vi "Read series.vi"(8 "error in (no error)":errorcluster, 11 "InovanceModbusTcp in":refnum<class "DeltaTcp.lvclass">) -> (0 "error out":errorcluster, 2 "series":i32(ring)=2 items=["DVP", "AS"], 3 "InovanceModbusTcp out":refnum<class "DeltaTcp.lvclass">)   [LabVIEW 2020, in "HslCommunication.lvlib" / "DeltaTcp.lvclass"]
uses:
  DeltaTcp.lvclass
  DeltaTcp.lvclass/DeltaTcp.ctl
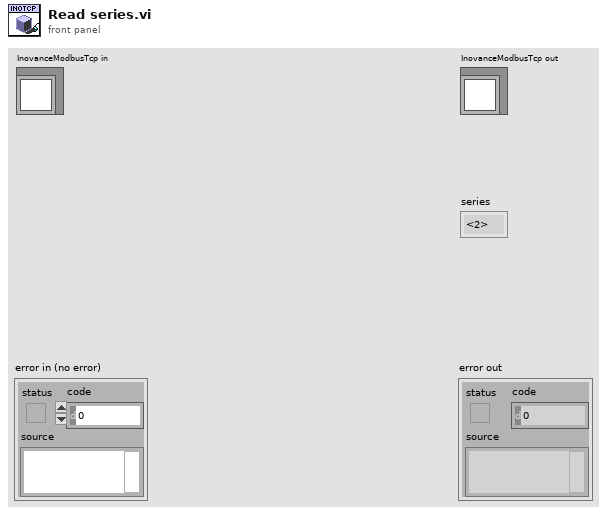
[diagram p1: front panel]
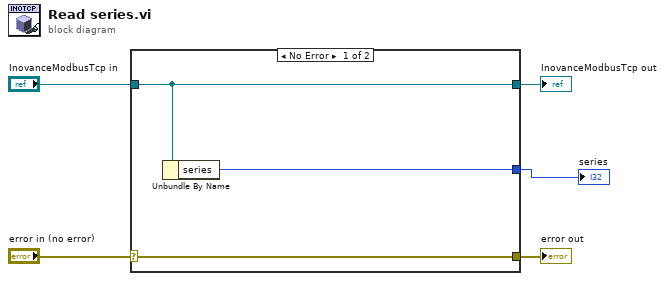
[diagram p0: block diagram]
diagram:
  n1 = case shown="No Error" "error in (no error)" {
    selector: "error in (no error)" -> [w8 w9]
    tunnel: [w8 w9] -> w4
    tunnel: [w7 w10] -> w2
    tunnel: "InovanceModbusTcp in" -> [w7 w10]
    tunnel: [w6 _] -> w1
    frame No Error {
      n2 = Unbundle By Name(w7) -> ("series"=w6:i32)
    }
    frame Error {
    }
  }
  "error out" <- w4
  "InovanceModbusTcp out" <- w2
  "series" <- w1
